vi "Set-Image-offset-x.vi"(8 "error in (no error)":errorcluster, 9 "Offset X in":i32, 10 "Image width":i32, 11 "Camera in":refnum<class "Camera.lvclass">) -> (0 "error out":errorcluster, 1 "Offset X":i32, 3 "Camera out":refnum<class "Camera.lvclass">)   [LabVIEW 2013, in "CameraVision.lvlib" / "Camera.lvclass"]
uses:
  Camera.lvclass
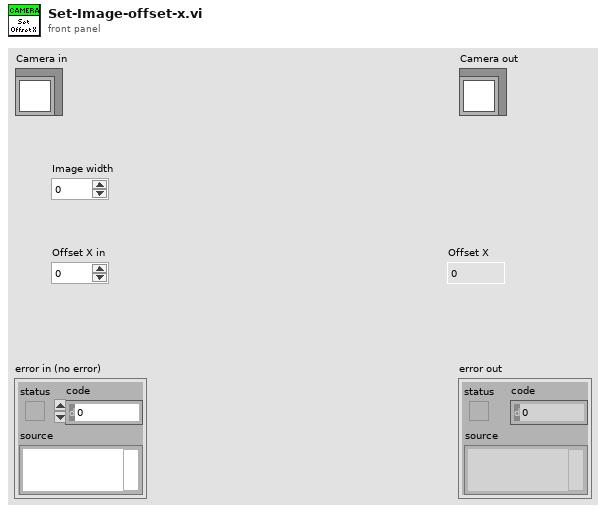
[diagram p1: front panel]
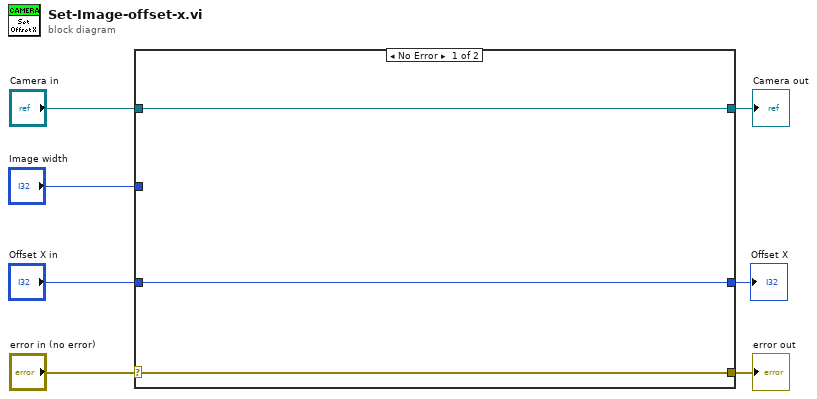
[diagram p0: block diagram]
diagram:
  n1 = case shown="No Error" "error in (no error)" {
    selector: "error in (no error)" -> [w9 w13]
    tunnel: [w9 w13] -> w6
    tunnel: [w10 w12] -> w4
    tunnel: "Camera in" -> [w10 w12]
    tunnel: [w8 w11] -> w2
    tunnel: "Offset X in" -> [w8 w11]
    tunnel: "Image width" -> [_ _]
    frame No Error {
    }
    frame Error {
    }
  }
  "error out" <- w6
  "Camera out" <- w4
  "Offset X" <- w2
